vi "setup_lc_rk.vi"(0 "didian":string, 4 "shuoming":string, 7 "zc_luodi_num":string, 9 "yw":string, 10 "id":string) -> (2 "error":errorcluster caption="error out 2")   [LabVIEW 2017, in "Lib_code.lvlib"]
uses:
  Lib_code.lvlib
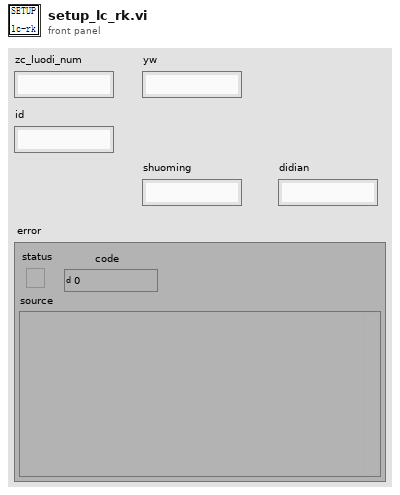
[diagram p1: front panel]
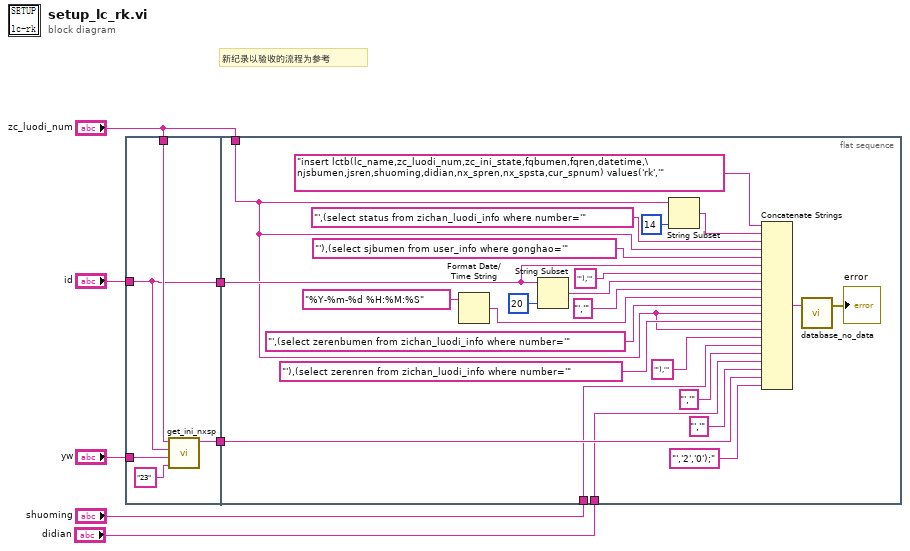
[diagram p0: block diagram]
diagram:
  # "新纪录以验收的流程为参考"
  n1 = flat-sequence {
    tunnel: "id" -> [w10]
    tunnel: [w10] -> w6
    tunnel: [w12] -> w5
    tunnel: "yw" -> [w9]
    tunnel: "zc_luodi_num" -> [w11]
    tunnel: w6 -> [w27]
    tunnel: w5 -> [w26]
    tunnel: "zc_luodi_num" -> [w13]
    tunnel: "shuoming" -> [w23]
    tunnel: "didian" -> [w18]
    frame #0 {
      n2 = call "get_ini_nxsp.vi"("juese"="23", "yw"=w9, "id"=w10, "zc_luodi_num"=w11) -> ("sp_gonghao"=w12:string)  [unwired: 7 in]
    }
    frame #1 {
      n3 = Format Date/Time String(time format string (%c)="%Y-%m-%d %H:%M:%S" ("时间格式字符串(%c)")) -> (date/time string=w16:string)  [unwired: 2 in]
      n4 = String Subset(string=w27, length (rest)=20 ("长度（剩余）")) -> (substring=w29:string)  [unwired: 1 in]
      n5 = String Subset(string=w13, length (rest)=14 ("长度（剩余）")) -> (substring=w34:string)  [unwired: 1 in]
      n6 = Concatenate Strings("insert lctb(lc_name,zc_luodi_num,zc_ini_state,fqbumen,fqren,datetime,\njsbumen,jsren,shuoming,didian,nx_spren,nx_spsta,cur_spnum) values('rk','" ("格式字符串"), w34, "',(select status from zichan_luodi_info where number='" ("字符串"), w13, "'),(select sjbumen from user_info where gonghao='" ("字符串"), w27, "'),'" ("字符串"), w29, "','" ("字符串"), w16, "',(select zerenbumen from zichan_luodi_info where number='" ("字符串"), w13, "'),(select zerenren from zichan_luodi_info where number='" ("字符串"), w13, "'),'" ("字符串"), w23, "','" ("字符串"), w18, "','" ("字符串"), w26, "','2','0');" ("字符串")) -> (w21:string)
      n7 = call "database_no_data.vi"("input"=w21) -> ("error"=→"error":errorcluster)  [unwired: 2 in]
    }
  }
